vi "Init Elevator.vi"() -> (2 "Slave Out":T1={"DeviceStatus"={"status"=FALSE, "code"=0, "source"=""}, "Type"=enum."PWM", "PWM"={"PWM Channel"=enum."Invalid", "DeadBand"={"Name"="", "maxPositivePwm"=0, "minPositivePwm"=0, "centerPwm"=0, "maxNegativePwm"=0, "minNegativePwm"=0, "angularRange"=0}}, "CAN"={"Device Number"=0, "SetOutput VI Ref"=variant(refnum<vi> refnum), "GetOutput VI Ref"=variant(refnum<vi> refnum), "Enable VI Ref"=variant(refnum<vi> refnum), "Disable VI Ref"=variant(refnum<vi> refnum), "Data"=variant}, "Invert"=FALSE, "DIO PWM"={"PWM \"Enable\" Channel"=enum."Invalid", "DIOChannel"=enum."Invalid", "PWM Rate"=0.0}}, 3 "Master Out":T1={"DeviceStatus"={"status"=FALSE, "code"=0, "source"=""}, "Type"=enum."PWM", "PWM"={"PWM Channel"=enum."Invalid", "DeadBand"={"Name"="", "maxPositivePwm"=0, "minPositivePwm"=0, "centerPwm"=0, "maxNegativePwm"=0, "minNegativePwm"=0, "angularRange"=0}}, "CAN"={"Device Number"=0, "SetOutput VI Ref"=variant(refnum<vi> refnum), "GetOutput VI Ref"=variant(refnum<vi> refnum), "Enable VI Ref"=variant(refnum<vi> refnum), "Disable VI Ref"=variant(refnum<vi> refnum), "Data"=variant}, "Invert"=FALSE, "DIO PWM"={"PWM \"Enable\" Channel"=enum."Invalid", "DIOChannel"=enum."Invalid", "PWM Rate"=0.0}})   [LabVIEW 2018]
uses:
  <vilib>/Rock Robotics/WPI/ThirdParty/REV Robotics/SPARK MAX/Typedef/Spark MAX Smart Motion Parameters.ctl
  <vilib>/Rock Robotics/WPI/MotorControl/WPI_MotorControlDeviceRef.ctl
  <vilib>/Rock Robotics/WPI/MotorControl/WPI_MotorControlType.ctl
  <vilib>/Rock Robotics/SystemInterfaces/DIO/FPGA_DIOPWMChannel.ctl
  <vilib>/Rock Robotics/WPI/PWM/WPI_PWMDeadband.ctl
  <vilib>/Rock Robotics/SystemInterfaces/DIO/FPGA_DIOChannel.ctl
  <vilib>/Rock Robotics/WPI/ThirdParty/REV Robotics/SPARK MAX/Typedef/Spark MAX Motor Type.ctl
  <vilib>/Rock Robotics/WPI/ThirdParty/REV Robotics/SPARK MAX/Typedef/Spark MAX Idle Mode.ctl
panel:
  in  "PID Constants":T6={"P Gain"=0.0, "I Gain"=0.0, "D Gain"=0.0, "F Gain"=0.0, "I Zone"=0.0, "Min Output"=-1.0, "Max Output"=1.0}
  in  "Smart Motion Parameters":T7
  in  "Invert":bool
  in  "Primary Current Limit":dbl=80.0
  in  "Slave Device Number":u8=8
  in  "Master Device Number":u8=7
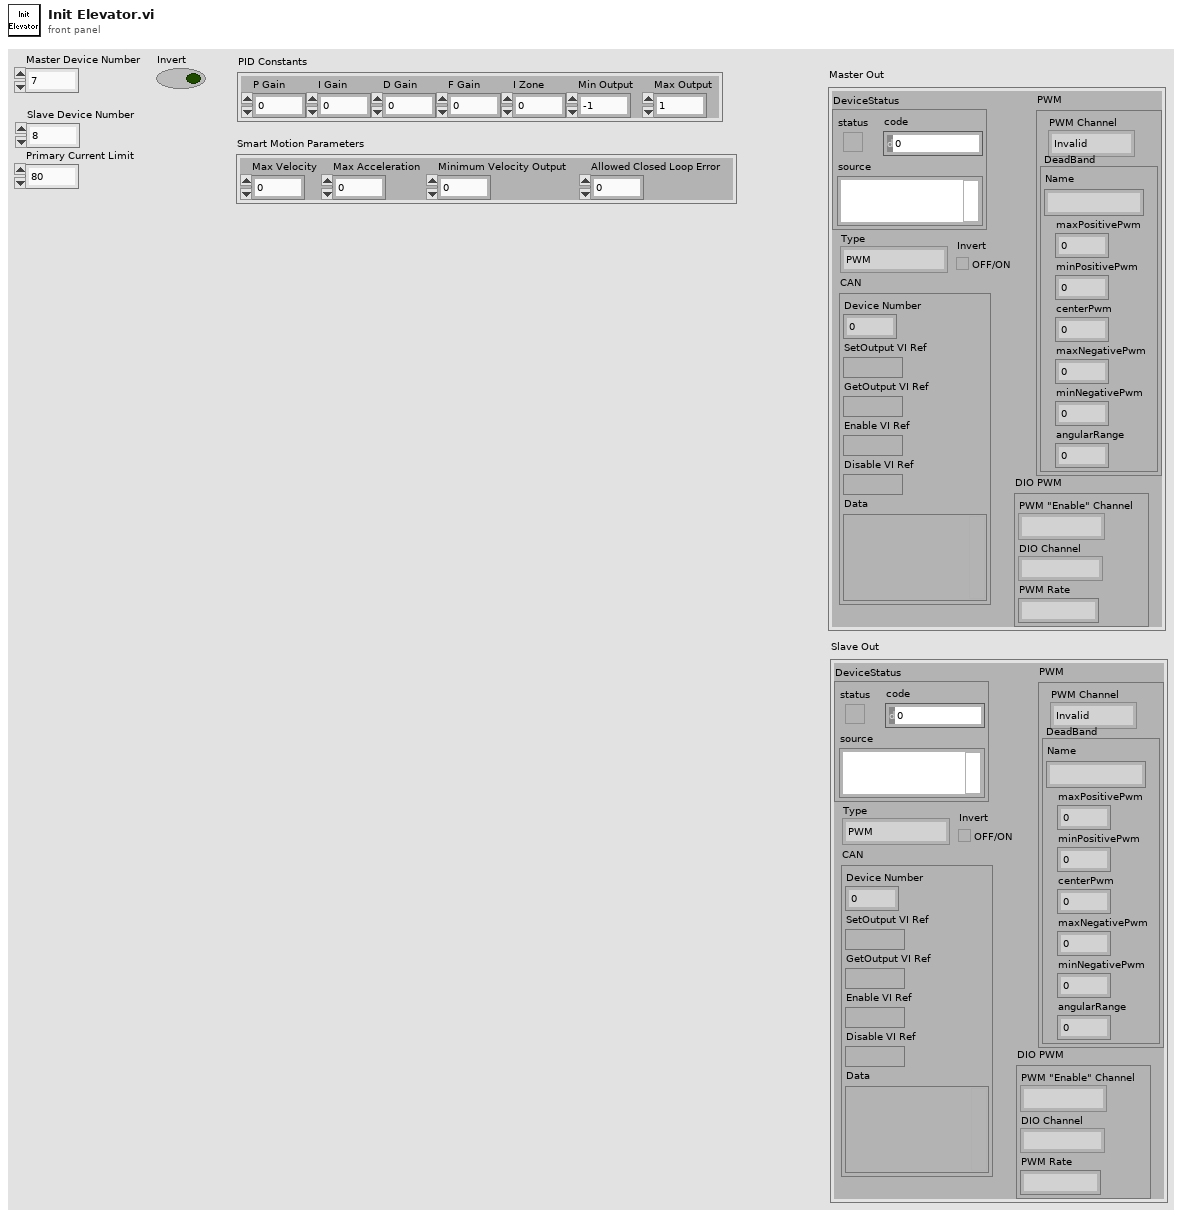
[diagram p1: front panel]
types:
  T1 = typedef "WPI_MotorControlDeviceRef.ctl" = cluster{"DeviceStatus":errorcluster, "Type":T2, "PWM":cluster{"PWM Channel":T3, "DeadBand":T4}, "CAN":cluster{"Device Number":u8, "SetOutput VI Ref":variant, "GetOutput VI Ref":variant, "Enable VI Ref":variant, "Disable VI Ref":variant, "Data":variant}, "Invert":bool, "DIO PWM":cluster{"PWM \"Enable\" Channel":T3, "DIOChannel":T5, "PWM Rate":dbl}}
  T2 = typedef "WPI_MotorControlType.ctl" = enum16{"PWM", "CAN", "DIO PWM"}
  T3 = typedef "FPGA_DIOPWMChannel.ctl" = enum8{"PWM 0", "PWM 1", "PWM 2", "PWM 3", "PWM 4", "PWM 5", "PWM 6", "PWM 7", "PWM 8", "PWM 9", "PWM MXP 0", "PWM MXP 1", "PWM MXP 2", "PWM MXP 3", "PWM MXP 4", "PWM MXP 5", "PWM MXP 6", "PWM MXP 7", "PWM MXP 8", "PWM MXP 9", "Invalid"}
  T4 = typedef "WPI_PWMDeadband.ctl" = cluster{"Name":string, "maxPositivePwm":i32, "minPositivePwm":i32, "centerPwm":i32, "maxNegativePwm":i32, "minNegativePwm":i32, "angularRange":u16}
  T5 = typedef "FPGA_DIOChannel.ctl" = enum8{"DIO 0", "DIO 1", "DIO 2", "DIO 3", "DIO 4", "DIO 5", "DIO 6", "DIO 7", "DIO 8", "DIO 9", "DIO MXP 0", "DIO MXP 1", "DIO MXP 2", "DIO MXP 3", "DIO MXP 4", "DIO MXP 5", "DIO MXP 6", "DIO MXP 7", "DIO MXP 8", "DIO MXP 9", "DIO MXP 10", "DIO MXP 11", "DIO MXP 12", "DIO MXP 13", "DIO MXP 14", "DIO MXP 15", "SPI Port CS1", "SPI Port CS2", "SPI Port CS3", "SPI Port MISO", "SPI Port MOSI", "Invalid"}
  T6 = cluster{"P Gain":dbl, "I Gain":dbl, "D Gain":dbl, "F Gain":dbl, "I Zone":dbl, "Min Output":dbl, "Max Output":dbl}
  T7 = typedef "Spark MAX Smart Motion Parameters.ctl" = cluster{"Max Velocity":dbl, "Max Acceleration":dbl, "Minimum Velocity Output":dbl, "Allowed Closed Loop Error":dbl}
  T8 = typedef "Spark MAX Idle Mode.ctl" = enum16{"Coast", "Brake"}
  T9 = typedef "Spark MAX Motor Type.ctl" = enum16{"Brushed", "Brushless"}
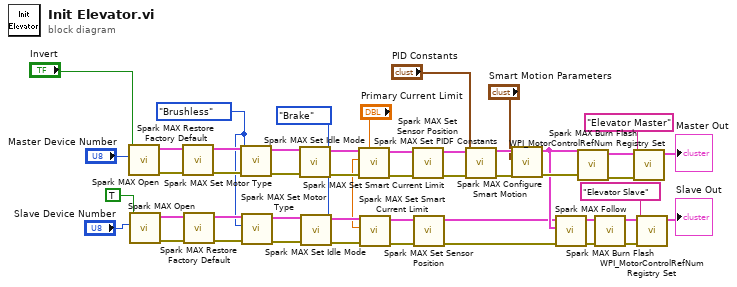
[diagram p0: block diagram]
diagram:
  w21 = Spark_MAX_Idle_Mode."Brake" ("Idle Mode")
  w22 = Spark_MAX_Motor_Type."Brushless" ("Enum")
  n1 = call <vilib>:"Spark MAX Open.vi"("Invert"="Invert", "Device Number"="Master Device Number") -> ("error out"=w46:errorcluster, "MotorControlDeviceRef"=w45:T1)  [unwired: 8 in]
  n2 = call <vilib>:"Spark MAX Open.vi"("Invert"=TRUE, "Device Number"="Slave Device Number") -> ("error out"=w33:errorcluster, "MotorControlDeviceRef"=w32:T1)  [unwired: 8 in]
  n3 = call <vilib>:"Spark MAX Restore Factory Default.vi"("error in"=w46, "MotorControlDeviceRef"=w45) -> ("error out"=w44:errorcluster, "MotorControlDeviceRef"=w43:T1)  [unwired: 8 in]
  n4 = call <vilib>:"Spark MAX Restore Factory Default.vi"("error in"=w33, "MotorControlDeviceRef"=w32) -> ("error out"=w31:errorcluster, "MotorControlDeviceRef"=w30:T1)  [unwired: 8 in]
  n5 = call <vilib>:"Spark MAX Set Motor Type.vi"("error in (no error)"=w44, "Enum"=w22, "MotorControlDevRef"=w43) -> ("error out"=w42:errorcluster, "MotorControlDeviceRef"=w41:T1)  [unwired: 7 in]
  n6 = call <vilib>:"Spark MAX Set Motor Type.vi"("error in (no error)"=w31, "Enum"=w22, "MotorControlDevRef"=w30) -> ("error out"=w29:errorcluster, "MotorControlDeviceRef"=w28:T1)  [unwired: 7 in]
  n7 = call <vilib>:"Spark MAX Set Idle Mode.vi"("error in (no error)"=w42, "Idle Mode"=w21, "MotorControlDeviceRef in"=w41) -> ("error out"=w40:errorcluster, "MotorControlDeviceRef out"=w39:T1)  [unwired: 7 in]
  n8 = call <vilib>:"Spark MAX Set Idle Mode.vi"("error in (no error)"=w29, "Idle Mode"=w21, "MotorControlDeviceRef in"=w28) -> ("error out"=w27:errorcluster, "MotorControlDeviceRef out"=w26:T1)  [unwired: 7 in]
  n9 = call <vilib>:"Spark MAX Set Smart Current Limit.vi"("error in (no error)"=w40, "Primay Current Limit (80A)"="Primary Current Limit", "MotorControlDeviceRef in"=w39) -> ("error out"=w38:errorcluster, "MotorControlDeviceRef out"=w37:T1)  [unwired: 7 in]
  n10 = call <vilib>:"Spark MAX Set Smart Current Limit.vi"("error in (no error)"=w27, "Primay Current Limit (80A)"="Primary Current Limit", "MotorControlDeviceRef in"=w26) -> ("error out"=w25:errorcluster, "MotorControlDeviceRef out"=w24:T1)  [unwired: 7 in]
  n11 = call <vilib>:"Spark MAX Set Sensor Position.vi"("error in"=w38, "MotorControlDeviceRef"=w37) -> ("error out"=w35:errorcluster, "MotorControlDeviceRef"=w34:T1)  [unwired: 8 in]
  n12 = call <vilib>:"Spark MAX Set Sensor Position.vi"("error in"=w25, "MotorControlDeviceRef"=w24) -> ("error out"=w4:errorcluster, "MotorControlDeviceRef"=w5:T1)  [unwired: 8 in]
  n13 = call <vilib>:"Spark MAX Set PIDF Constants.vi"("error in"=w35, "PID Constants"="PID Constants", "MotorControlDeviceRef"=w34) -> ("error out"=w16:errorcluster, "MotorControlDeviceRef"=w19:T1)  [unwired: 7 in]
  n14 = call <vilib>:"Spark MAX Configure Smart Motion.vi"("error in"=w16, "Smart Motion Parameters"="Smart Motion Parameters", "MotorControlDeviceRef"=w19) -> ("error out"=w15:errorcluster, "MotorControlDeviceRef"=w6:T1)  [unwired: 7 in]
  n15 = call <vilib>:"Spark MAX Follow.vi"("error in (no error)"=w4, "Master Controller"=w6, "MotorControlDeviceRef"=w5) -> ("error out"=w10:errorcluster, "MotorControlDeviceRef"=w9:T1)  [unwired: 7 in]
  n16 = call <vilib>:"Spark MAX Burn Flash.vi"("error in"=w15, "MotorControlDeviceRef"=w6) -> ("error out"=w14:errorcluster, "MotorControlDeviceRef"=w13:T1)  [unwired: 8 in]
  n17 = call <vilib>:"Spark MAX Burn Flash.vi"("error in"=w10, "MotorControlDeviceRef"=w9) -> ("error out"=w7:errorcluster, "MotorControlDeviceRef"=w8:T1)  [unwired: 8 in]
  n18 = call <vilib>:"WPI_MotorControlRefNum Registry Set.vi"("error in (no error)"=w14, "refnum name"="Elevator Master", "MotorControlDevRef"=w13) -> ("MotorControlDevRef"=→"Master Out":T1)  [unwired: 7 in, 1 out]
  n19 = call <vilib>:"WPI_MotorControlRefNum Registry Set.vi"("error in (no error)"=w7, "refnum name"="Elevator Slave", "MotorControlDevRef"=w8) -> ("MotorControlDevRef"=→"Slave Out":T1)  [unwired: 7 in, 1 out]
